vi "grabMoveReinit.vi"(4 "End position mm":dbl, 5 "acquire?":bool, 6 "Start position mm":dbl, 7 "microscope event queue":refnum<queue>, 8 "Step Number in":i32, 9 "image event queue":refnum<queue>, 10 "Step size microns (discrete)":dbl) -> (3 "Step Number out":i32)   [LabVIEW 2012, in "Microscope.lvclass"]
uses:
  classes/Microscope.lvclass
  typedefs/ImageEvent.ctl
  typedefs/MicroscopeEvent.ctl
  variables/GlobalUI.vi
  sequences/partial_stop_sequence.vi
  sequences/discrete_acquire_sequence.vi
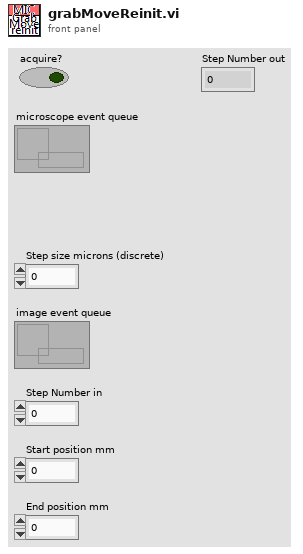
[diagram p1: front panel]
types:
  T1 = typedef "ImageEvent.ctl" = enum16{"i.Wait", "i.Acquire", "i.InitImageData", "i.ReinitImageData", "i.ReinitImageParams", "i.PreAcquire", "i.PostAcquire", "i.ClearData"}
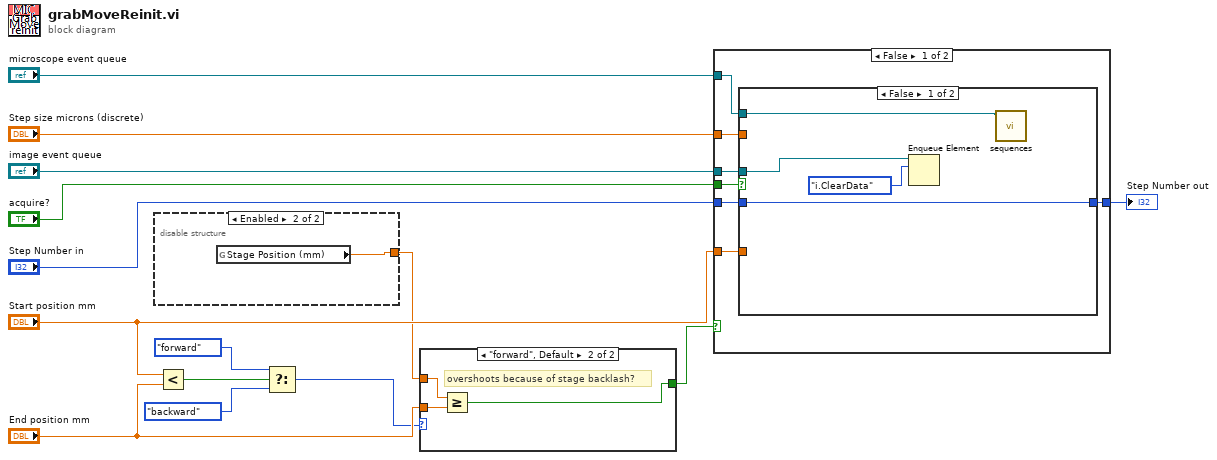
[diagram p0: block diagram]
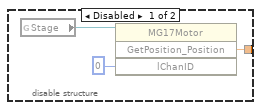
[diagram p2: hidden frame]
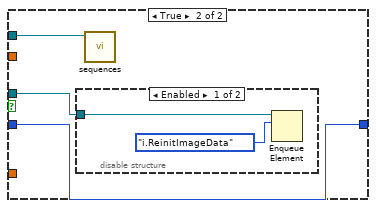
[diagram p3: hidden frame]
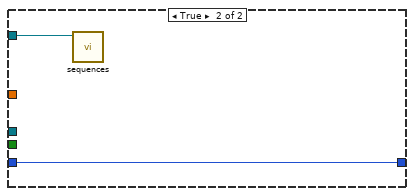
[diagram p5: hidden frame]
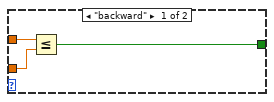
[diagram p6: hidden frame]
diagram:
  n1 = disable-structure shown="Enabled" {
    disable-tunnel: [w16 w18] -> w3
    frame Disabled {
      n2 = global read "GlobalUI.vi" "Stage"() -> (w15:refnum<k7>)
      n3 = invoke class="MG17Motor" method="GetPosition_Position"(reference=w15, "lChanID"=0) -> ("GetPosition_Position"=w16:sgl)  [unwired: 2 in, 3 out]
    }
    frame Enabled {
      n4 = global read "GlobalUI.vi" "Stage Position (mm)"() -> (w18:dbl)
    }
  }
  n5 = Less?(x="Start position mm", y="End position mm") -> (x < y?=w5:bool)
  n6 = Select(t=enum16{"", "forward", "backward"}."forward", s=w5, f=enum16{"", "forward", "backward"}."backward") -> (s? t:f=w2:enum16{"", "forward", "backward"})
  n7 = case shown="\"forward\", Default" w2 {
    tunnel: [w21 w24] -> w8
    tunnel: w3 -> [w20 w22]
    tunnel: "End position mm" -> [w19 w23]
    frame "backward" {
      n8 = Less Or Equal?(x=w20, y=w19) -> (x <= y?=w21:bool)
    }
    frame "forward", Default {
      # "overshoots because of stage backlash?"
      n9 = Greater Or Equal?(x=w22, y=w23) -> (x >= y?=w24:bool)
    }
  }
  n10 = case shown="False" w8 {
    tunnel: "microscope event queue" -> [w31 w41]
    tunnel: "Step Number in" -> [w30 w42]
    tunnel: "Step size microns (discrete)" -> [w29 _]
    tunnel: "Start position mm" -> [w28 _]
    tunnel: [w27 w42] -> w12
    tunnel: "image event queue" -> [w26 _]
    tunnel: "acquire?" -> [w25 _]
    frame False {
      n11 = case shown="False" w25 {
        tunnel: w31 -> [w32 w36]
        tunnel: w30 -> [w35 w38]
        tunnel: w29 -> [_ _]
        tunnel: w28 -> [_ _]
        tunnel: [w35 w38] -> w27
        tunnel: w26 -> [w34 w37]
        frame False {
          n12 = Enqueue Element(queue=w34, element=ImageEvent."i.ClearData") -> ()  [unwired: 2 in, 3 out]
          n13 = call-poly "sequences.vi"("Queue in"=w32) -> ()  [unwired: 9 in, 2 out]
        }
        frame True {
          n14 = disable-structure shown="Enabled" {
            disable-tunnel: w37 -> [w40 _]
            frame Enabled {
              n15 = Enqueue Element(queue=w40, element=ImageEvent."i.ReinitImageData") -> ()  [unwired: 2 in, 3 out]
            }
            frame Disabled {
            }
          }
          n16 = call-poly "sequences.vi"("Queue in"=w36) -> ()  [unwired: 11 in]
        }
      }
    }
    frame True {
      n17 = call-poly "sequences.vi"("Queue in"=w41) -> ()  [unwired: 9 in, 2 out]
    }
  }
  "Step Number out" <- w12
